vi "RMS_meas (SubVI).vi"(8 "error in (no error)":errorcluster, 10 "freq_search":dbl[](array[numeric]), 11 "Array 3":waveform(dbl)[](array[waveform])) -> (0 "error out":errorcluster, 2 "RMS_Array":dbl[](array[numeric]), 3 "Freq_Array":dbl[](array[numeric]))   [LabVIEW 2017]
uses:
  <vilib>/Analysis/4window.llb/windowTd.ctl
  <vilib>/measure/maspectr.llb/FFT Spectrum (Mag-Phase) for N Chan.vi
  <vilib>/measure/NI_MAPro.lvlib
  <vilib>/Analysis/NI_AALPro.lvlib
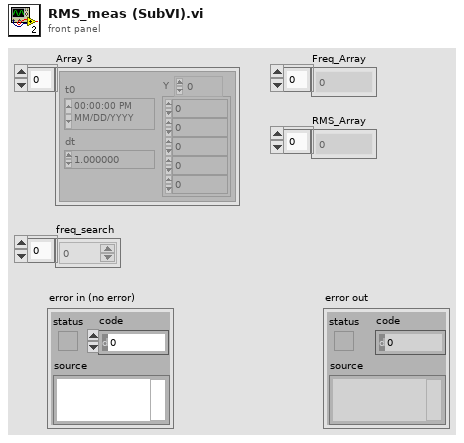
[diagram p1: front panel]
types:
  T1 = cluster{"averaging mode":enum16{"No averaging", "Vector averaging", "RMS averaging", "Peak hold"}, "weighting mode":enum16{"Linear", "Exponential"}, "number of averages":u32}
  T2 = typedef "NI_AALPro.lvlib/windowTd.ctl" = u32
  T3 = cluster{"dB On (F)":bool, "unwrap phase (F)":bool, "convert to degree (F)":bool}
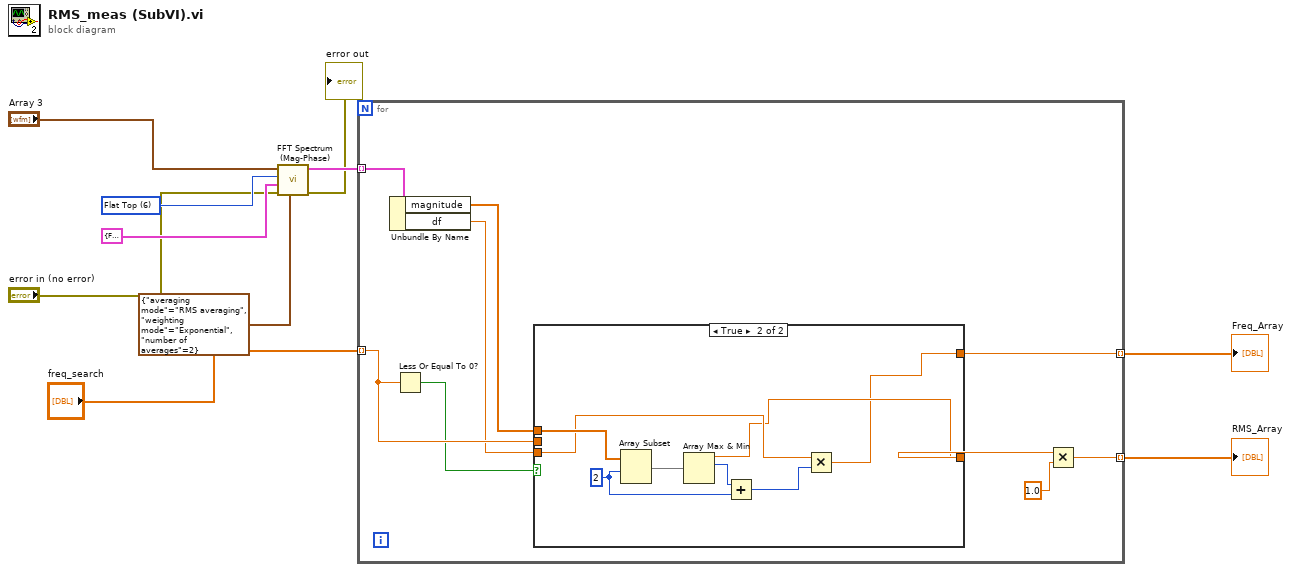
[diagram p0: block diagram]
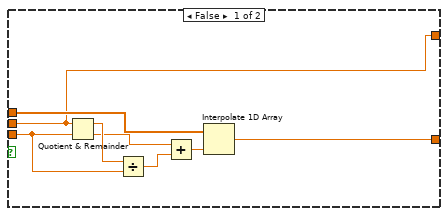
[diagram p2: hidden frame]
diagram:
  w5 = T2 6 items=["Rectangle"=0, "Hanning"=1, "Hamming"=2, "Blackman-Harris"=3, "Exact Blackman"=4, "Blackman"=5, "Flat Top"=6, "4 Term B-Harris "=7, "7 Term B-Harris"=8, "Low Sidelobe"=9, "Blackman Nuttall"=11, "Triangle"=30, "Bartlett-Hanning"=31, "Bohman"=32, "Parzen"=33, "Welch"=34, "Kaiser"=60, "Dolph-Chebyshev"=61, "Gaussian"=62] ("window")
  n1 = call-poly <vilib>:"FFT Spectrum (Mag-Phase).vi"("averaging parameters"=T1 {"averaging mode"=enum."RMS averaging", "weighting mode"=enum."Exponential", "number of averages"=2}, "error in (no error)"="error in (no error)", "view"=T3 {"dB On (F)"=FALSE, "unwrap phase (F)"=FALSE, "convert to degree (F)"=FALSE}, "window"=w5, "time signals"="Array 3") -> ("error out"=→"error out":errorcluster, "magnitudes"=w4:cluster{"f0":dbl, "df":dbl, "magnitude":dbl[]}[])  [unwired: 2 in, 3 out]
  n2 = for {
    tunnel: w4 -> [w18] mode=indexing
    tunnel: [w15] -> w8 mode=indexing
    tunnel: "freq_search" -> [w17] mode=indexing
    tunnel: [w11] -> w10 mode=indexing
    n3 = Unbundle By Name(w18) -> ("magnitude"=w14:dbl[], "df"=w13:dbl)
    n4 = Less Or Equal To 0?(x=w17) -> (x <= 0?=w12:bool)
    n5 = case shown="True" w12 {
      tunnel: w17 -> [w20 _]
      tunnel: [w23 w29] -> w16
      tunnel: w14 -> [w22 w31]
      tunnel: w13 -> [w21 w30]
      tunnel: [w20 w28] -> w11
      frame False {
        n6 = Quotient & Remainder(x=w20, y=w21) -> (x-y*floor(x/y)=w27:dbl, floor(x/y)=w25:dbl)
        n7 = Divide(x=w27, y=w21) -> (x/y=w26:dbl)
        n8 = Add(x=w25, y=w26) -> (x+y=w24:dbl)
        n9 = Interpolate 1D Array(1:w24, 2:w22) -> (0:w23:dbl)
      }
      frame True {
        w32 = 2 ("index")
        n10 = Array Subset(array=w31, index=w32) -> (w35:dbl[])  [unwired: 1 in]
        n11 = Array Max & Min(array=w35) -> (max value=w29:dbl, max index (indices)=w34:i32)  [unwired: 2 out]
        n12 = Add(x=w34, y=w32) -> (x+y=w33:i32)
        n13 = Multiply(x=w30, y=w33) -> (x*y=w28:dbl)
      }
    }
    n14 = Multiply(x=w16, y=1.0 ("sqrt(x)")) -> (x*y=w15:dbl)
  }
  "Freq_Array" <- w10
  "RMS_Array" <- w8
